vi "poly_normalise_DBL.vi"(6 "mode (max)":enum16{"max", "rms"}(ring), 10 "input":dbl[](array[numeric]) format="%#_13g") -> (2 "output":dbl[](array[numeric]) format="%#_13g")   [LabVIEW 2015]
uses:
  <vilib>/Analysis/baseanly.llb/Mean (DBL).vi
  <vilib>/Analysis/NI_AALBase.lvlib
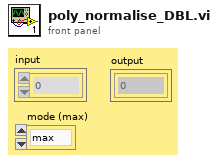
[diagram p1: front panel]
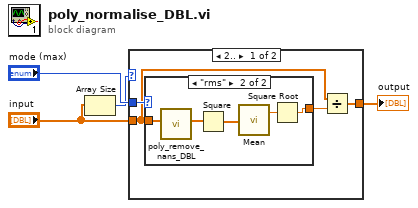
[diagram p0: block diagram]
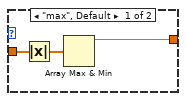
[diagram p2: hidden frame]
diagram:
  n1 = Array Size(array="input") -> (size(s)=w1:i32)
  n2 = case shown="2.." w1 {
    tunnel: "mode (max)" -> [w8 _]
    tunnel: "input" -> [w6 w17]
    tunnel: [w7 w17] -> w3
    frame 2.. {
      n3 = case shown="\"rms\"" w8 {
        tunnel: w6 -> [w10 w13]
        tunnel: [w9 w14] -> w5
        frame "max", Default {
          n4 = Absolute Value(x=w10) -> (abs(x)=w11:dbl[])
          n5 = Array Max & Min(array=w11) -> (max value=w9:dbl)  [unwired: 3 out]
        }
        frame "rms" {
          n6 = call "poly_remove_nans_DBL.vi"("input"=w13) -> ("output"=w12:dbl[])  [unwired: 9 in, 1 out]
          n7 = Square(x=w12) -> (x^2=w16:dbl[])
          n8 = call-poly <vilib>:"Mean.vi"("X"=w16) -> ("mean"=w15:dbl)  [unwired: 1 out]
          n9 = Square Root(x=w15) -> (sqrt(x)=w14:dbl)
        }
      }
      n10 = Divide(x=w6, y=w5) -> (x/y=w7:dbl[])
    }
    frame ..1 {
    }
  }
  "output" <- w3
